vi "Make_Target_Wavelength_Table.vi"(0 ".NET Reference in":refnum<k24>, 5 "startwave":dbl, 7 "endwave":dbl, 9 "targetdatastep":dbl, 11 "error in (no error)":errorcluster) -> (4 "Reference out":refnum<k24>, 15 "error out":errorcluster)   [LabVIEW 2017]
doc: "Make rescaling wavelength step table"
uses:
  D:/test/ILSTS/LV_IL_Sample/DLL/STSProcess.dll
  DLL/STSProcess.dll
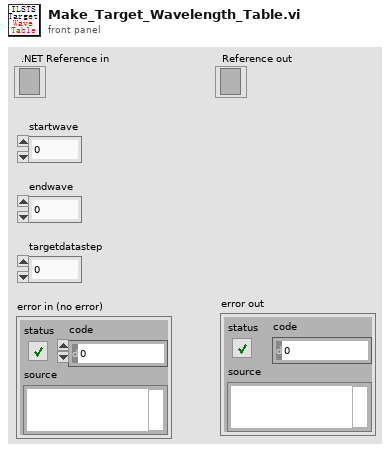
[diagram p1: front panel]
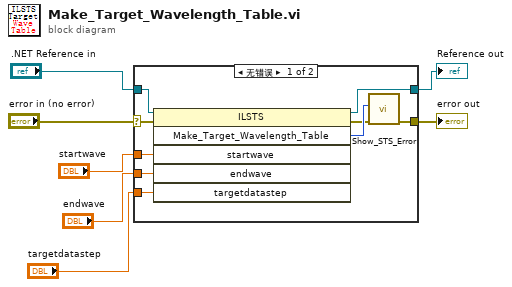
[diagram p0: block diagram]
diagram:
  n1 = case shown="无错误" "error in (no error)" {
    selector: "error in (no error)" -> [w14 w18]
    tunnel: ".NET Reference in" -> [w16 w17]
    tunnel: [w15 w17] -> w6
    tunnel: [w11 w18] -> w4
    tunnel: "startwave" -> [w10 _]
    tunnel: "endwave" -> [w9 _]
    tunnel: "targetdatastep" -> [w8 _]
    frame No Error {
      n2 = invoke on="调用节点" class="ILSTS" method="Make_Target_Wavelength_Table"(reference=w16, error in=w14, "startwave"=w10, "endwave"=w9, "targetdatastep"=w8) -> (reference out=w15:refnum<k24>, error out=w12:errorcluster, "Make_Target_Wavelength_Table"=w13:i32)  [unwired: 1 in, 3 out]
      n3 = call "Show_STS_Error.vi"("error in (no error)"=w12, "Error"=w13) -> ("error out"=w11:errorcluster)  [unwired: 9 in]
    }
    frame Error {
    }
  }
  "error out" <- w4
  "Reference out" <- w6
